vi "AmpTest.vi"() -> ()   [LabVIEW 2020]
uses:
  Realization/PI650 VoltageAmp/PI650 VoltageAmp.lvclass
panel:
  in  "DC Offset":cluster{"Channel (CH1)":u32, "Offset (128)":u32}={"Channel (CH1)"=1, "Offset (128)"=128} {"Channel (CH1)" items=["CH1"=1, "CH2"=2, "CH3"=3, "CH4"=4, "CH5"=5]}
  in  "Gain":cluster{"Channel (CH1)":u32, "Gain (x1)":u32}={"Channel (CH1)"=1, "Gain (x1)"=1} {"Channel (CH1)" items=["CH1"=1, "CH2"=2, "CH3"=3, "CH4"=4, "CH5"=5]; "Gain (x1)" items=["x1"=1, "x2"=2, "x5"=3, "x7"=4, "x10"=5, "x14"=6, "x20"=7]}
  out "DC Offset":variant
  out "error out":errorcluster
  out "Status":variant
  out "Info":variant
  out "Result":variant
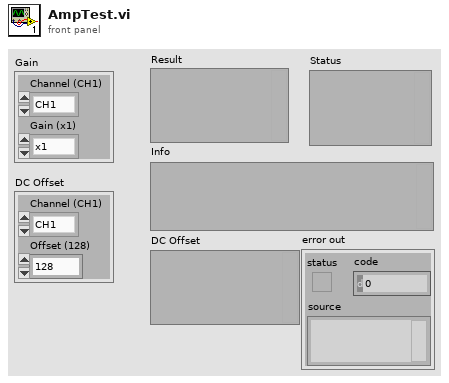
[diagram p1: front panel]
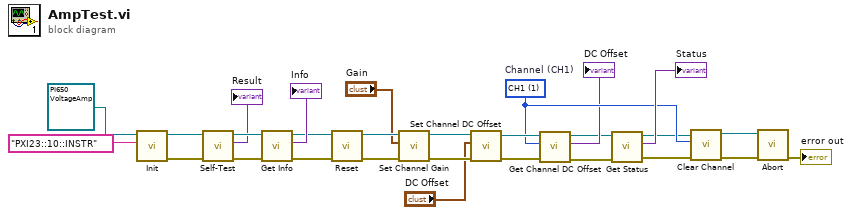
[diagram p0: block diagram]
diagram:
  w8 = u32 1 items=["CH1"=1, "CH2"=2, "CH3"=3, "CH4"=4, "CH5"=5]  # Channel (CH1)
  n1 = call-dynamic "Init.vi"("Params"="PXI23::10::INSTR", "PI650 VoltageAmp in"=refnum<class "PI650 VoltageAmp.lvclass"> refnum) -> ("error out"=w24:errorcluster, "PI650 VoltageAmp out"=w28:refnum<class "PI650 VoltageAmp.lvclass">)  [unwired: 8 in]
  n2 = call-dynamic "Self-Test.vi"("error in (no error)"=w24, "PI650 VoltageAmp in"=w28) -> ("error out"=w23:errorcluster, "Result"=→"Result":variant, "PI650 VoltageAmp out"=w27:refnum<class "PI650 VoltageAmp.lvclass">)  [unwired: 7 in]
  n3 = call-dynamic "Get Info.vi"("error in (no error)"=w23, "PI650 VoltageAmp in"=w27) -> ("error out"=w7:errorcluster, "Info"=→"Info":variant, "PI650 VoltageAmp out"=w6:refnum<class "PI650 VoltageAmp.lvclass">)  [unwired: 7 in]
  n4 = call-dynamic "Reset.vi"("error in (no error)"=w7, "PI650 VoltageAmp in"=w6) -> ("error out"=w22:errorcluster, "PI650 VoltageAmp out"=w26:refnum<class "PI650 VoltageAmp.lvclass">)  [unwired: 8 in]
  n5 = call-dynamic "Set Channel Gain.vi"("error in (no error)"=w22, "Params"="Gain", "PI650 VoltageAmp in"=w26) -> ("error out"=w14:errorcluster, "PI650 VoltageAmp out"=w13:refnum<class "PI650 VoltageAmp.lvclass">)  [unwired: 7 in]
  n6 = call-dynamic "Set Channel DC Offset.vi"("error in (no error)"=w14, "Params"="DC Offset", "PI650 VoltageAmp in"=w13) -> ("error out"=w12:errorcluster, "PI650 VoltageAmp out"=w11:refnum<class "PI650 VoltageAmp.lvclass">)  [unwired: 7 in]
  n7 = call-dynamic "Get Channel DC Offset.vi"("error in (no error)"=w12, "Params"=w8, "PI650 VoltageAmp in"=w11) -> ("error out"=w4:errorcluster, "DC Offset"=→"DC Offset":variant, "PI650 VoltageAmp out"=w3:refnum<class "PI650 VoltageAmp.lvclass">)  [unwired: 6 in]
  n8 = call-dynamic "Get Status.vi"("error in (no error)"=w4, "PI650 VoltageAmp in"=w3) -> ("error out"=w1:errorcluster, "Status"=→"Status":variant, "PI650 VoltageAmp out"=w2:refnum<class "PI650 VoltageAmp.lvclass">)  [unwired: 7 in]
  n9 = call-dynamic "Clear Channel.vi"("error in (no error)"=w1, "Params"=w8, "PI650 VoltageAmp in"=w2) -> ("error out"=w21:errorcluster, "PI650 VoltageAmp out"=w25:refnum<class "PI650 VoltageAmp.lvclass">)  [unwired: 7 in]
  n10 = call-dynamic "Abort.vi"("error in (no error)"=w21, "PI650 VoltageAmp in"=w25) -> ("error out"=→"error out":errorcluster)  [unwired: 8 in, 1 out]
